vi "FTW-Connector-Ask.vi"(0 "FTW Actor Connector":refnum<class "FTW-ActorConnector.lvclass">, 5 "Request Header":string, 7 "Request Body":string, 9 "Timeout":i32=100 format="%dmsec", 11 "error in":errorcluster) -> (4 "FTW Actor Connector out":refnum<class "FTW-ActorConnector.lvclass">, 6 "Response Header":string, 8 "Response Body":string, 10 "Timed out?":bool, 14 "Roundtrip Time":dbl format="%.6fsec", 15 "error out":errorcluster)   [LabVIEW 2013, in "FTW-ActorConnector.lvclass"]
uses:
  FTW-ActorConnector.lvclass
  FTW-ActorConnector.lvclass/FTW-ActorConnector.ctl
  Endpoint/FTW-Endpoint.lvclass
panel:
  # "Inputs"
  # "Outputs"
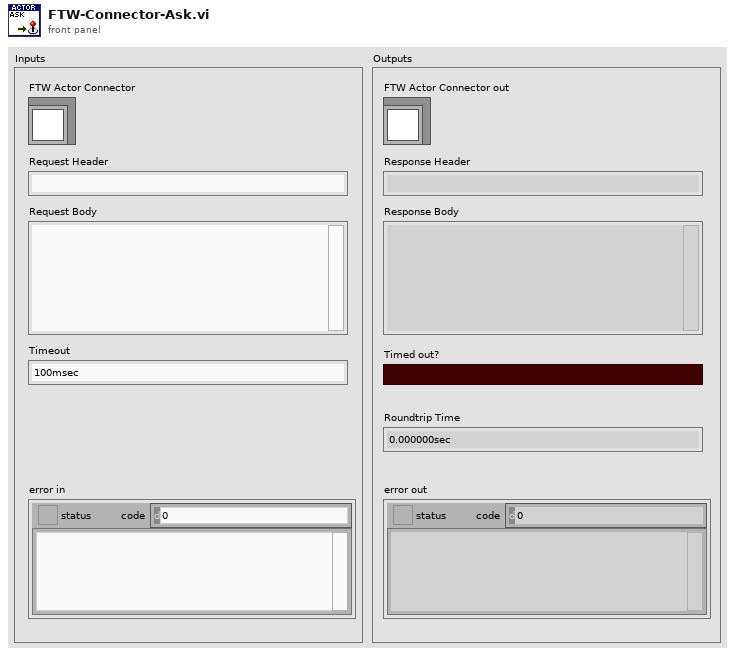
[diagram p1: front panel]
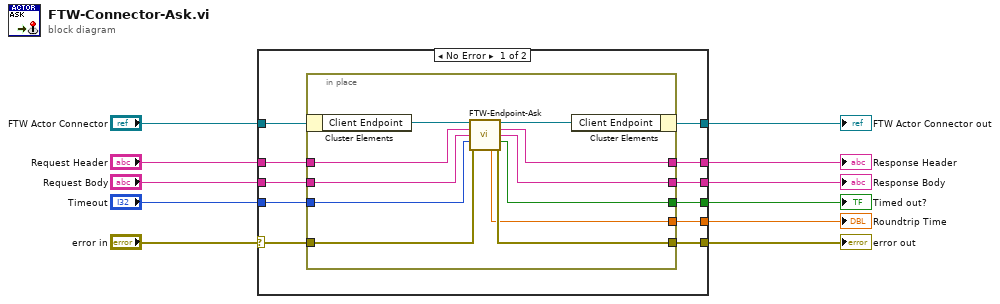
[diagram p0: block diagram]
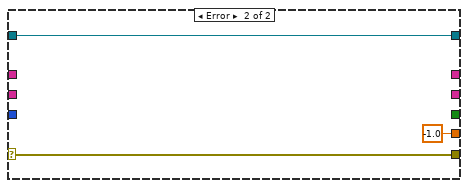
[diagram p2: hidden frame]
diagram:
  n1 = case shown="No Error" "error in" {
    selector: "error in" -> [w21 w36]
    tunnel: [w19 w36] -> w10
    tunnel: "FTW Actor Connector" -> [w22 w35]
    tunnel: [w20 w35] -> w8
    tunnel: "Request Header" -> [w18 _]
    tunnel: "Request Body" -> [w17 _]
    tunnel: [w16 _] -> w7
    tunnel: "Timeout" -> [w15 _]
    tunnel: [w14 _] -> w3
    tunnel: [w13 _] -> w2
    tunnel: [w12 -1.0 ("Roundtrip Time")] -> w1
    frame No Error {
      n2 = in-place {
        in-place-border: w21 -> [w33]
        in-place-border: [w32] -> w19
        in-place-border: w18 -> [w28]
        in-place-border: w17 -> [w27]
        in-place-border: [w29] -> w16
        in-place-border: w15 -> [w26]
        in-place-border: [w25] -> w14
        in-place-border: [w24] -> w13
        in-place-border: [w23] -> w12
        n3 = in-place-cluster #1(w22) -> ("Client Endpoint"=w31:refnum<class "FTW-Endpoint.lvclass">)
        n4 = call-dynamic "FTW-Endpoint-Ask.vi"("FTW Endpoint"=w31, "Request Header"=w28, "Request Body"=w27, "Timeout"=w26, "error in"=w33) -> ("FTW Endpoint out"=w30:refnum<class "FTW-Endpoint.lvclass">, "Response Header"=w25:string, "Response Body"=w24:string, "Timed out?"=w29:bool, "Roundtrip Time"=w23:dbl, "error out"=w32:errorcluster)  [unwired: 5 in]
        n5 = in-place-cluster #1("Client Endpoint"=w30) -> (w20:refnum<class "FTW-ActorConnector.lvclass">)
      }
    }
    frame Error {
    }
  }
  "error out" <- w10
  "FTW Actor Connector out" <- w8
  "Timed out?" <- w7
  "Response Header" <- w3
  "Response Body" <- w2
  "Roundtrip Time" <- w1
